vi "HiCCE_Display_v2.0.vi"() -> ()   [LabVIEW 2019]
panel:
  out "decimated array 2":u16[](array[numeric])
  out "decimated array":u16[](array[numeric])
  out "DEC_STATUS 2":u8[](array[numeric])
  in  "stop":bool
  out "Waveform Chart":u32[][](graph)
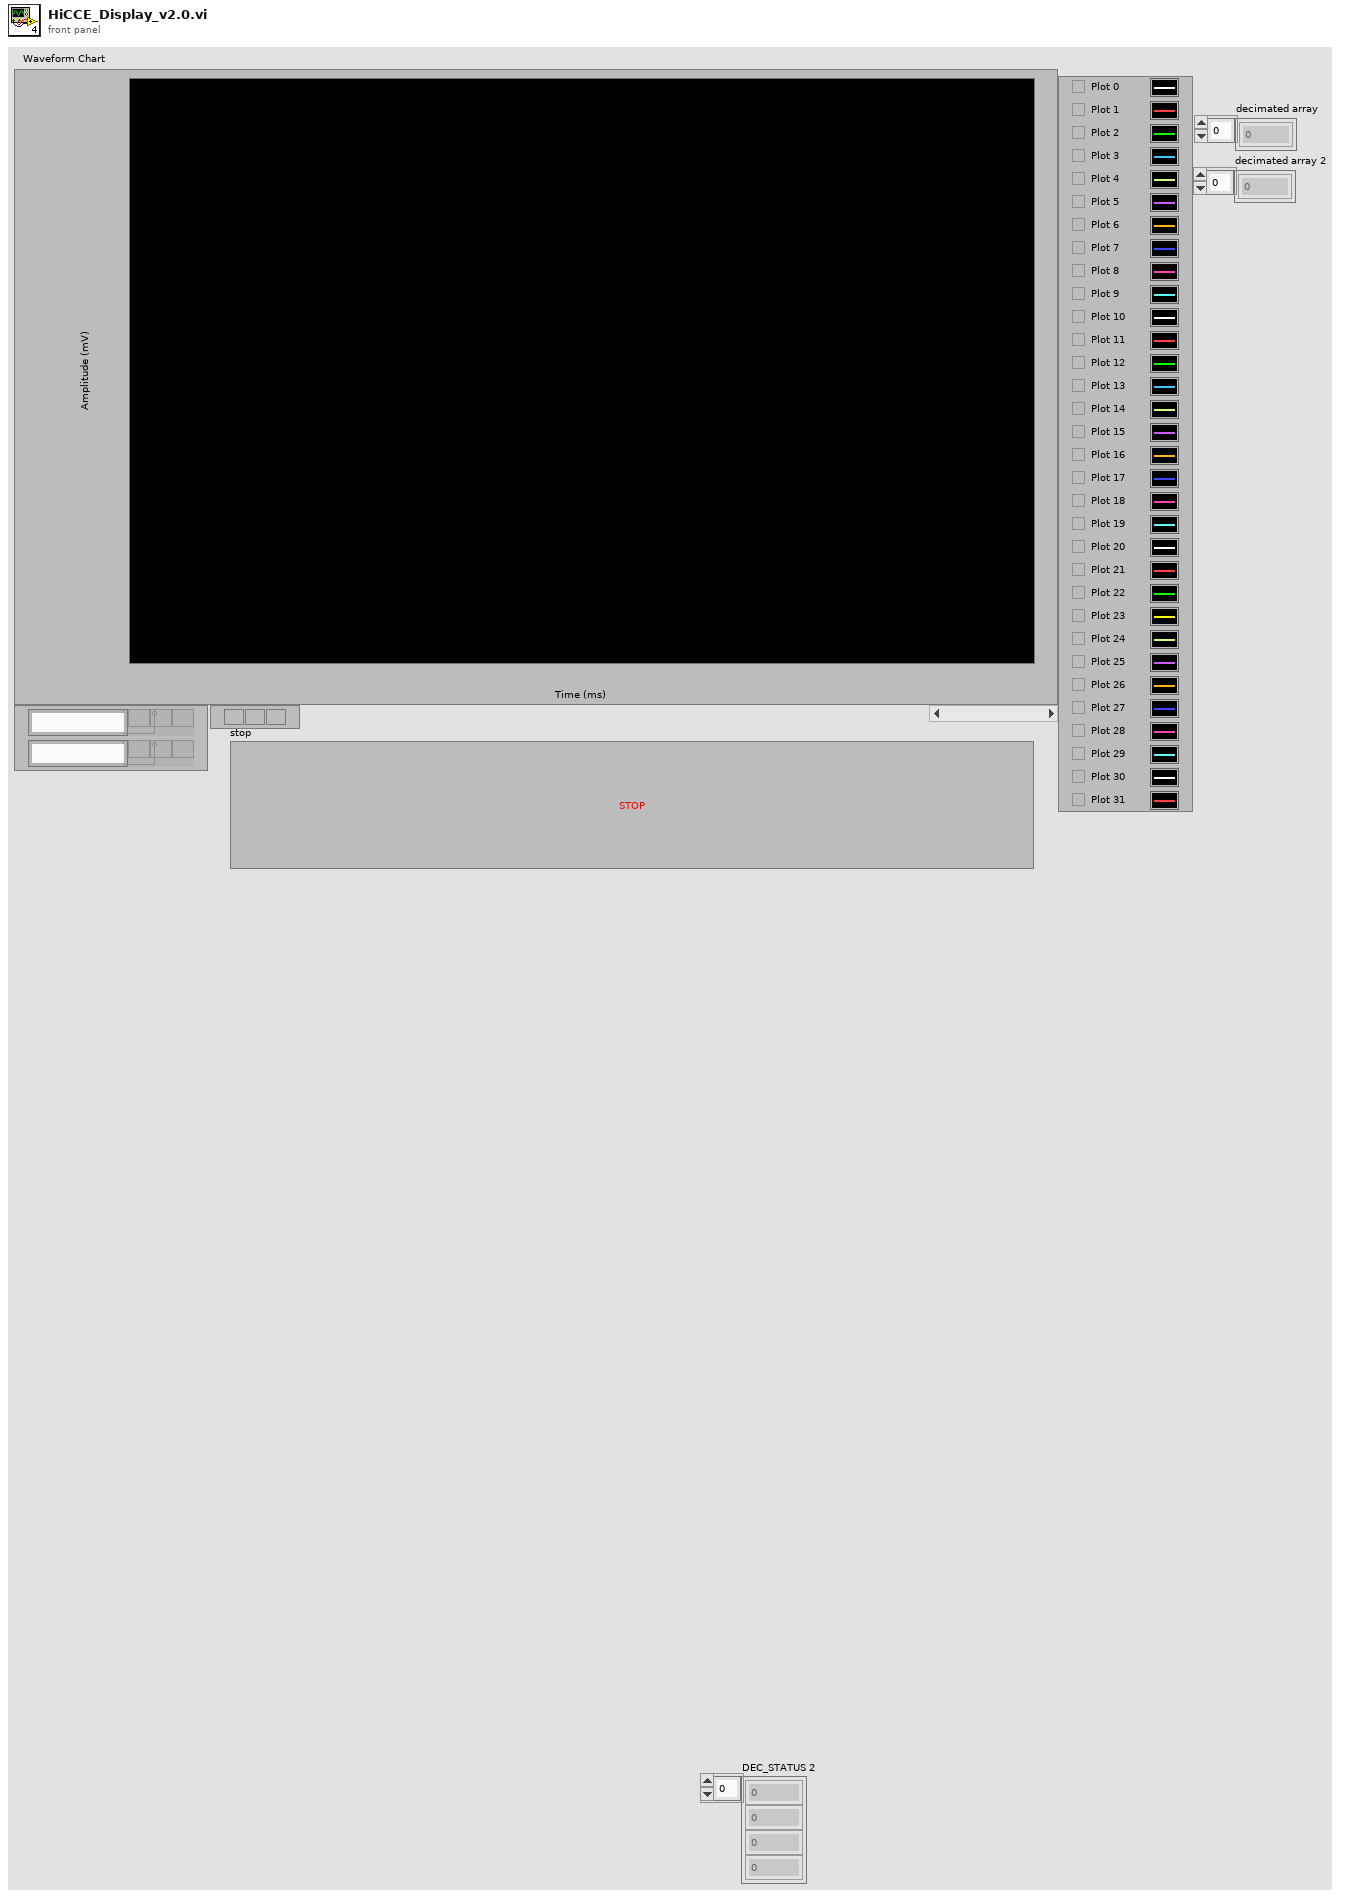
[diagram p1: front panel]
types:
  T1 = enum16{"big-endian, network order", "native, host order", "little-endian"}
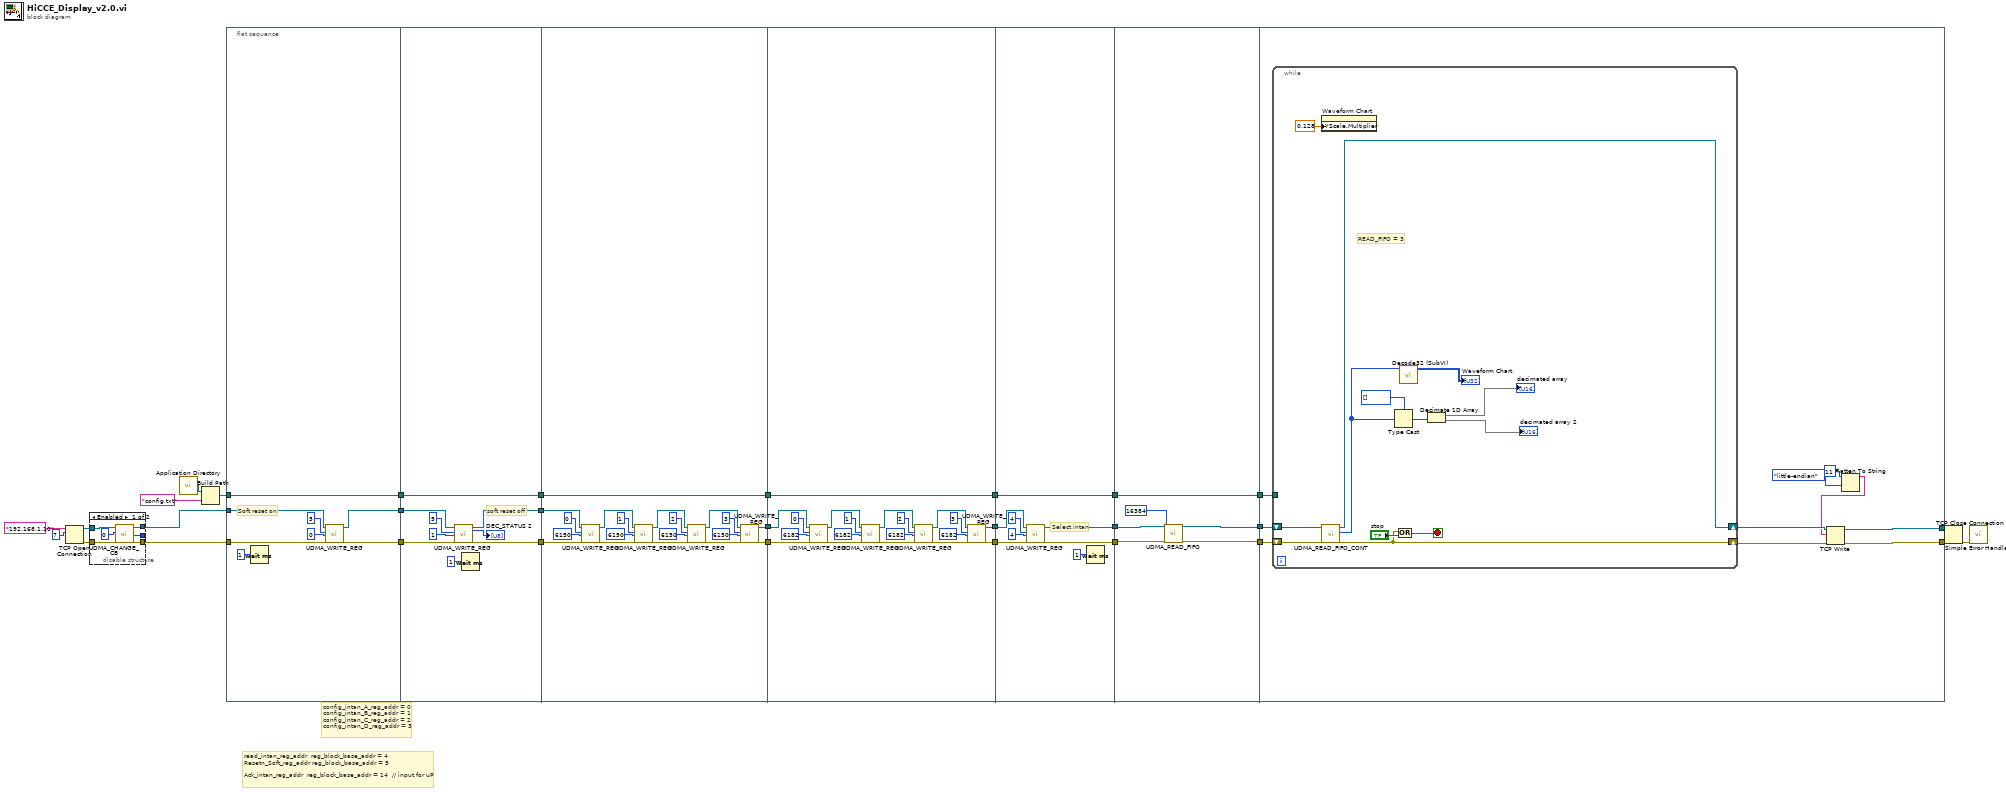
[diagram p0: block diagram]
diagram:
  # "read_intan_reg_addr\t\treg_block_base_addr = 4\nResetn_Soft_reg_addr\treg_block_base_addr = 5\n\nAck_intan_reg_addr\t\treg_block_base_addr = 14\t\t// input for uP"
  # "config_intan_A_reg_addr = 0\nconfig_intan_B_reg_addr = 1\nconfig_intan_C_reg_addr = 2\nconfig_intan_D_reg_addr = 3"
  n1 = TCP Open Connection(address="192.168.1.10", remote port or service name=u16 7) -> (connection ID=w12:refnum<k5>, error out=w11:errorcluster)  [unwired: 3 in]
  n2 = disable-structure shown="Enabled" {
    disable-tunnel: w12 -> [w36 w38]
    disable-tunnel: w11 -> [w35 w37]
    disable-tunnel: [w33 w38] -> w10
    disable-tunnel: [w32 w37] -> w9
    disable-tunnel: [w31 _] -> _
    frame Enabled {
      n3 = call "UDMA_CHANGE_CB.vi"("TCP Network Connection in"=w36, "CB_ID"=u32 0, "error in (no error)"=w35) -> ("TCP Network Connection out"=w33:refnum<k5>, "STATUS"=w31:u32, "error out"=w32:errorcluster)  [unwired: 14 in]
    }
    frame Disabled {
    }
  }
  n4 = call <vilib>:"Application Directory.vi"() -> ("Application Directory"=w25:path)
  n5 = Build Path(base path=w25, name or relative path="config.txt") -> (appended path=w23:path)
  n6 = flat-sequence {
    tunnel: w23 -> [w46]
    tunnel: [w46] -> w22
    tunnel: w10 -> [w44]
    tunnel: w9 -> [w43]
    tunnel: [w40] -> w20
    tunnel: [w39] -> w19
    tunnel: w22 -> [w55]
    tunnel: [w55] -> w21
    tunnel: w20 -> [w53]
    tunnel: w19 -> [w52]
    tunnel: [w48] -> w18
    tunnel: [w47] -> w17
    tunnel: [w74] -> w16
    tunnel: w21 -> [w74]
    tunnel: w18 -> [w62]
    tunnel: w17 -> [w61]
    tunnel: [w57] -> w14
    tunnel: [w56] -> w13
    tunnel: w16 -> [w93]
    tunnel: [w93] -> w15
    tunnel: w14 -> [w78]
    tunnel: w13 -> [w77]
    tunnel: [w76] -> w8
    tunnel: [w75] -> w7
    tunnel: [w95] -> w6
    tunnel: [w94] -> w4
    tunnel: w15 -> [w101]
    tunnel: [w101] -> w2
    tunnel: w8 -> [w99]
    tunnel: w7 -> [w98]
    tunnel: w6 -> [w106]
    tunnel: [w105] -> w5
    tunnel: w4 -> [w103]
    tunnel: [w102] -> w3
    tunnel: w2 -> [w107]
    tunnel: [w107] -> w1
    tunnel: [w113] -> w28
    tunnel: [w112] -> w27
    tunnel: w5 -> [w117]
    tunnel: w3 -> [w116]
    tunnel: w1 -> [w111]
    frame #0 {
      # "Soft reset on"
      n7 = Wait (ms)(milliseconds to wait=u32 1) -> ()  [unwired: 1 out]
      n8 = call "UDMA_WRITE_REG.vi"("TCP Network Connection in"=w44, "REG"=u32 5, "DATA"=u32 0, "error in (no error)"=w43) -> ("TCP Network Connection out"=w40:refnum<k5>, "error out"=w39:errorcluster)  [unwired: 13 in, 1 out]
    }
    frame #1 {
      # "soft reset off"
      n9 = call "UDMA_WRITE_REG.vi"("TCP Network Connection in"=w53, "REG"=u32 5, "DATA"=u32 1, "error in (no error)"=w52) -> ("TCP Network Connection out"=w48:refnum<k5>, "DEC_STATUS"=→"DEC_STATUS 2":u8[], "error out"=w47:errorcluster)  [unwired: 13 in]
      n10 = Wait (ms)(milliseconds to wait=u32 1) -> ()  [unwired: 1 out]
    }
    frame #2 {
      n11 = call "UDMA_WRITE_REG.vi"("TCP Network Connection in"=w62, "REG"=u32 0, "DATA"=u32 6150, "error in (no error)"=w61) -> ("TCP Network Connection out"=w65:refnum<k5>, "error out"=w60:errorcluster)  [unwired: 13 in, 1 out]
      n12 = call "UDMA_WRITE_REG.vi"("TCP Network Connection in"=w65, "REG"=u32 1, "DATA"=u32 6150, "error in (no error)"=w60) -> ("TCP Network Connection out"=w64:refnum<k5>, "error out"=w59:errorcluster)  [unwired: 13 in, 1 out]
      n13 = call "UDMA_WRITE_REG.vi"("TCP Network Connection in"=w64, "REG"=u32 2, "DATA"=u32 6150, "error in (no error)"=w59) -> ("TCP Network Connection out"=w63:refnum<k5>, "error out"=w58:errorcluster)  [unwired: 13 in, 1 out]
      n14 = call "UDMA_WRITE_REG.vi"("TCP Network Connection in"=w63, "REG"=u32 3, "DATA"=u32 6150, "error in (no error)"=w58) -> ("TCP Network Connection out"=w57:refnum<k5>, "error out"=w56:errorcluster)  [unwired: 13 in, 1 out]
    }
    frame #3 {
      n15 = call "UDMA_WRITE_REG.vi"("TCP Network Connection in"=w78, "REG"=u32 0, "DATA"=u32 6182, "error in (no error)"=w77) -> ("TCP Network Connection out"=w84:refnum<k5>, "error out"=w81:errorcluster)  [unwired: 13 in, 1 out]
      n16 = call "UDMA_WRITE_REG.vi"("TCP Network Connection in"=w84, "REG"=u32 1, "DATA"=u32 6182, "error in (no error)"=w81) -> ("TCP Network Connection out"=w83:refnum<k5>, "error out"=w80:errorcluster)  [unwired: 13 in, 1 out]
      n17 = call "UDMA_WRITE_REG.vi"("TCP Network Connection in"=w83, "REG"=u32 2, "DATA"=u32 6182, "error in (no error)"=w80) -> ("TCP Network Connection out"=w82:refnum<k5>, "error out"=w79:errorcluster)  [unwired: 13 in, 1 out]
      n18 = call "UDMA_WRITE_REG.vi"("TCP Network Connection in"=w82, "REG"=u32 3, "DATA"=u32 6182, "error in (no error)"=w79) -> ("TCP Network Connection out"=w76:refnum<k5>, "error out"=w75:errorcluster)  [unwired: 13 in, 1 out]
    }
    frame #4 {
      # "Select intan"
      n19 = call "UDMA_WRITE_REG.vi"("TCP Network Connection in"=w99, "REG"=u32 4, "DATA"=u32 4, "error in (no error)"=w98) -> ("TCP Network Connection out"=w95:refnum<k5>, "error out"=w94:errorcluster)  [unwired: 13 in, 1 out]
      n20 = Wait (ms)(milliseconds to wait=u32 1) -> ()  [unwired: 1 out]
    }
    frame #5 {
      n21 = call "UDMA_READ_FIFO.vi"("TCP Network Connection in"=w106, "N"=u32 16384, "error in (no error)"=w103) -> ("TCP Network Connection out"=w105:refnum<k5>, "error out"=w102:errorcluster)  [unwired: 13 in, 2 out]
    }
    frame #6 {
      n22 = while {
        shift-right: [w124] -> w115
        shift-left: w117 -> [w126]
        shift-right: [w123] -> w114
        shift-left: w116 -> [w125]
        tunnel: w111 -> [_]
        stop <- w130 stop-if-true
        # "READ_FIFO = 3"
        n23 = property on="Waveform Chart" class="WFChart (strict)"("YScale.Multiplier"=0.128 ("Y Scale.Offset and Multiplier:Multiplier")) -> ()  [unwired: 2 in, 2 out]
        n24 = call "UDMA_READ_FIFO_CONT.vi"("TCP Network Connection in"=w126, "error in (no error)"=w125) -> ("TCP Network Connection out"=w124:refnum<k5>, "Oscilloscope"=w122:u32[], "error out"=w123:errorcluster)  [unwired: 14 in, 1 out]
        n25 = Type Cast(type=u16[] [], x=w122) -> (*(type *) &x=w120:u16[])
        n26 = Or(x=w123, y="stop") -> (x .or. y?=w130:bool)
        n27 = call "Decode32 (SubVI).vi"("Oscilloscope"=w122) -> ("Array"=→"Waveform Chart":u32[][])  [unwired: 10 in]
        n28 = Decimate 1D Array(w120) -> (→"decimated array":u16[], →"decimated array 2":u16[])
      }
      n29 = Flatten To String(anything=u32 11 ("element"), byte order (0:big-endian, network order)=T1."little-endian") -> (data string=w108:string)  [unwired: 2 in, 2 out]
      n30 = TCP Write(connection ID=w115, data in=w108, error in (no error)=w114) -> (connection ID out=w113:refnum<k5>, error out=w112:errorcluster)  [unwired: 1 in, 1 out]
    }
  }
  n31 = TCP Close Connection(connection ID=w28, error in (no error)=w27) -> (error out=w26:errorcluster)  [unwired: 1 in, 1 out]
  n32 = call <vilib>:"Simple Error Handler.vi"("error in (no error)"=w26) -> ()  [unwired: 4 in, 5 out]
